vi "Trigger and Read Meas.vi"(8 "error in (no error)":errorcluster, 9 "trigger mode (0:internal)":u16(ring) items=["internal - continuous trigger", "external - rear panel trigger with delay", "external - bus trigger with delay", "external - rear panel trigger", "external - bus trigger"], 11 "VISA resource name":refnum<visa-resource-name>) -> (0 "error out":errorcluster, 1 "unit":string, 2 "measurement":dbl format="%^.6e", 3 "VISA resource name out":refnum<visa-resource-name>)   [LabVIEW 2017, in "Fluke 8840.lvlib"]
doc: "This VI triggers the multimeter and reads the resulting measurement."
uses:
  Fluke 8840.lvlib
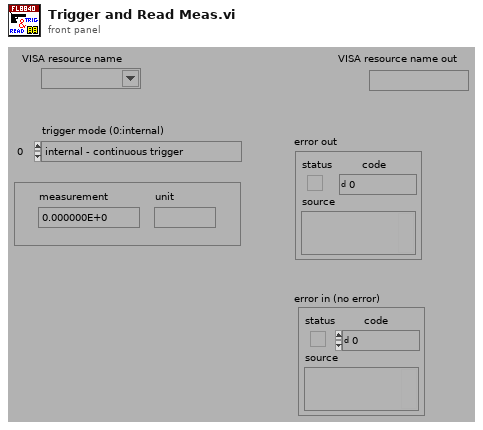
[diagram p1: front panel]
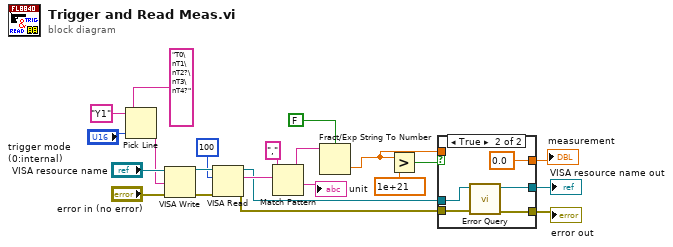
[diagram p0: block diagram]
diagram:
  n1 = Pick Line(string ("")="Y1", multi-line string="T0\nT1\nT2?\nT3\nT4?", line index="trigger mode (0:internal)") -> (output string=w18:string)
  n2 = VISA Write(VISA resource name="VISA resource name", write buffer=w18, error in (no error)="error in (no error)") -> (VISA resource name out=w16:refnum<visa-resource-name>, error out=w17:errorcluster)  [unwired: 1 out]
  n3 = VISA Read(VISA resource name=w16, byte count=100, error in (no error)=w17) -> (VISA resource name out=w4:refnum<visa-resource-name>, read buffer=w10:string, error out=w5:errorcluster)  [unwired: 1 out]
  n4 = Match Pattern(string=w10, regular expression=",") -> (before substring=w12:string, after substring=→"unit":string)  [unwired: 3 out]
  n5 = Fract/Exp String To Number(use system decimal point (T)=FALSE, string=w12) -> (number=w3:dbl)  [unwired: 3 out]
  n6 = Greater?(x=w3, y=1e+21) -> (0:w8:bool)
  n7 = case shown="True" w8 {
    tunnel: [w25 0.0] -> w2
    tunnel: [w24 w29] -> w7
    tunnel: [w23 w28] -> w6
    tunnel: w5 -> [w23 w27]
    tunnel: w4 -> [w24 w26]
    tunnel: w3 -> [w25 _]
    frame False {
    }
    frame True {
      n8 = call "Error Query.vi"("error in (no error)"=w27, "VISA resource name"=w26) -> ("error out"=w28:errorcluster, "VISA resource name out"=w29:refnum<visa-resource-name>)  [unwired: 1 in, 7 out]
    }
  }
  "error out" <- w6
  "VISA resource name out" <- w7
  "measurement" <- w2
